vi "Analyze.vi"(0 "Analyze Fluence in":refnum<class "Analyze Fluence.lvclass">, 1 "Create Overlay?":bool, 5 "Image in":T1, 7 "Parameters in":variant, 9 "Results in":variant, 11 "error in (no error)":errorcluster) -> (4 "Analyze Fluence out":refnum<class "Analyze Fluence.lvclass">, 6 "Image out":T1, 8 "Parameters out":variant, 10 "Results out":variant, 15 "error out":errorcluster)   [LabVIEW 2009, in "Analyze.lvlib" / "Analyze Fluence.lvclass"]
doc: "In Variant Attributes to provide:\nEnergy: Energy in J\nROI: Image Display ROI Deskriptor\n\nOut Variant Attributes:\nFluence Infos: Array of Fluence Info.ctl\nMax Fluence: Maximal detected Fluence in J/cm^2"
uses:
  Analyze Fluence.lvclass
  <vilib>/vision/Image Controls.llb/IMAQ Image.ctl
  Analyze BaseClass/Analyze BaseClass.lvclass
  Analyze Fluence.lvclass/Analyze Fluence.ctl
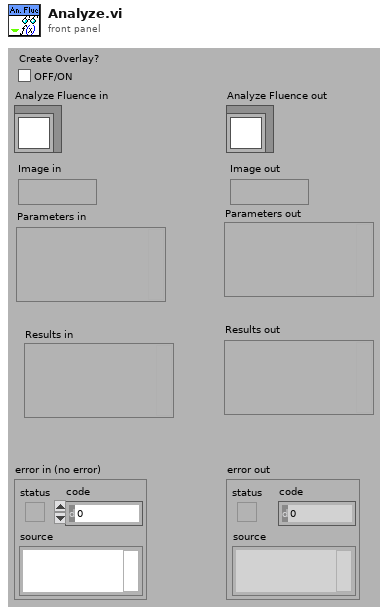
[diagram p1: front panel]
types:
  T1 = typedef "IMAQ Image.ctl" = refnum<image>
  T2 = typedef "Analyze.lvlib/Analyze Fluence.lvclass/Fluence Info.ctl" = cluster{"Fluence J/cm^2":dbl, "Energy in Area":dbl, "max value":i64, "Max fluence area":cluster{"Left":i32, "Top":i32, "Right":i32, "Bottom":i32}}
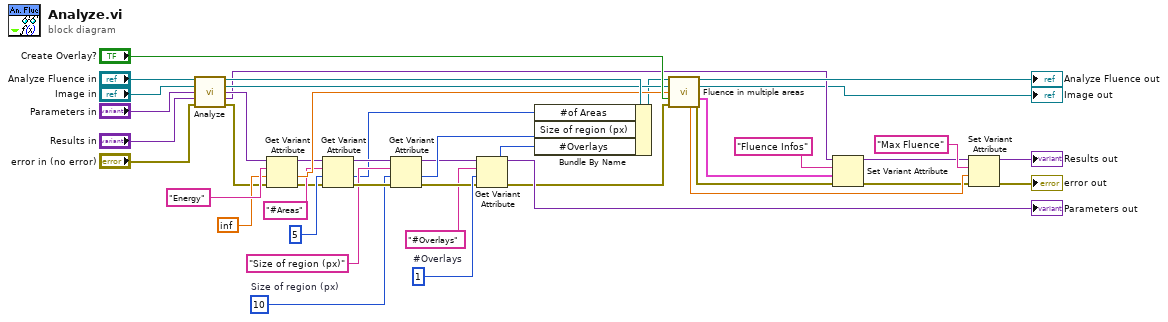
[diagram p0: block diagram]
diagram:
  w8 = 10  # Size of region (px)
  w7 = 1  # #Overlays
  n1 = call-parent "Analyze.vi"("Analyze BaseClass in"="Analyze Fluence in", "Image in"="Image in", "Parameters"="Parameters in", "Results in"="Results in", "error in (no error)"="error in (no error)") -> ("Analyze BaseClass out"=w29:refnum<class "Analyze Fluence.lvclass">, "Image out"=w27:T1, "Parameters out"=w25:variant, "Results"=w23:variant, "error out"=w21:errorcluster)  [unwired: 6 in]
  n2 = Get Variant Attribute(Variant=w25, name="Energy", default value (empty Variant)=inf, error in=w21) -> (duplicate Variant=w16:variant, value=w20:dbl, error out=w15:errorcluster)  [unwired: 1 out]
  n3 = Get Variant Attribute(Variant=w16, name="#Areas", default value (empty Variant)=5, error in=w15) -> (duplicate Variant=w14:variant, value=w9:i32, error out=w13:errorcluster)  [unwired: 1 out]
  n4 = Get Variant Attribute(Variant=w14, name="Size of region (px)", default value (empty Variant)=w8, error in=w13) -> (duplicate Variant=w6:variant, value=w10:i32, error out=w3:errorcluster)  [unwired: 1 out]
  n5 = Get Variant Attribute(Variant=w6, name="#Overlays", default value (empty Variant)=w7, error in=w3) -> (duplicate Variant=→"Parameters out":variant, value=w2:i32, error out=w4:errorcluster)  [unwired: 1 out]
  n6 = Bundle By Name(cluster=w29, "#of Areas"=w9, "Size of region (px)"=w10, "#Overlays"=w2) -> (w11:refnum<class "Analyze Fluence.lvclass">)
  n7 = call "Fluence in multiple areas.vi"("Analyze Fluence in"=w11, "Image in"=w27, "Energy"=w20, "Create Overlay(T)?"="Create Overlay?", "error in (no error)"=w4) -> ("Analyze Fluence out"=→"Analyze Fluence out":refnum<class "Analyze Fluence.lvclass">, "Image Dst Out"=→"Image out":T1, "Max Fluence J/cm^2"=w41:dbl, "fluence infos"=w34:T2[], "error out"=w37:errorcluster)  [unwired: 6 in]
  n8 = Set Variant Attribute(Variant=w23, name="Fluence Infos", value=w34, error in=w37) -> (Variant out=w35:variant, error out=w36:errorcluster)  [unwired: 1 out]
  n9 = Set Variant Attribute(Variant=w35, name="Max Fluence", value=w41, error in=w36) -> (Variant out=→"Results out":variant, error out=→"error out":errorcluster)  [unwired: 1 out]
